vi "testInvokeMethod.vi"() -> ()   [LabVIEW 2017]
panel:
  out "The result":i32
  out "pID":string
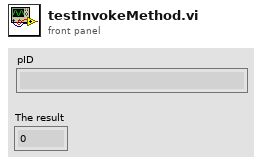
[diagram p1: front panel]
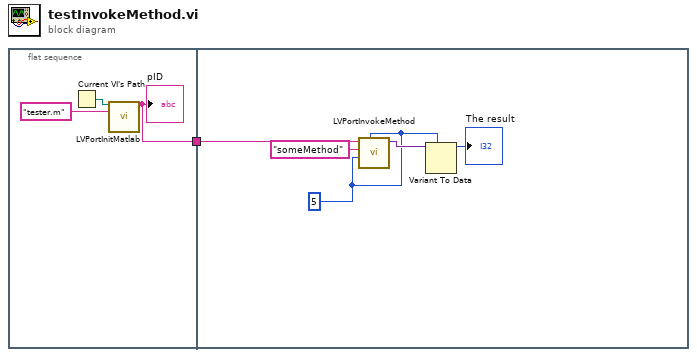
[diagram p0: block diagram]
diagram:
  n1 = flat-sequence {
    tunnel: [w2] -> w1
    tunnel: w1 -> [w9]
    frame #0 {
      n2 = Current VI's Path() -> (path=w4:path)
      n3 = call "LVPortInitMatlab.vi"("Working directory or VI Path"=w4, "Code file name"="tester.m") -> ("ID"=w2:string)  [unwired: 12 in, 1 out]
      "pID" <- w2
    }
    frame #1 {
      w6 = 5
      n4 = call "LVPortInvokeMethod.vi"("Result Type or Value to update (if any)"=w6, "Arguments (if nameless array then multi arguments)"=w6, "Method Name"="someMethod", "pID"=w9) -> ("Result (if any)"=w7:variant)  [unwired: 5 in, 2 out]
      n5 = Variant To Data(type=w6, Variant=w7) -> (data=→"The result":i32)  [unwired: 1 in, 1 out]
    }
  }
